vi "Test_Resize_Greyscale.vi"(8 "error in (no error)":errorcluster, 11 "Test Case In":refnum<class "Image.lvclass">) -> (0 "error out":errorcluster, 3 "Test Case Out":refnum<class "Image.lvclass">)   [LabVIEW 2020, in "g_ar_toolkit.test.lvlib" / "Image.lvclass"]
uses:
  Image.lvclass
  Image.lvclass/Image.ctl
  g_ar_toolkit.image/g_ar_toolkit.image.lvlib
  g_ar_toolkit.image/Image Size (Fixed).ctl
  g_ar_toolkit.image/CreateEmptyImageGreyscale.vi
  g_ar_toolkit.image/Interpolation Mode.ctl
  g_ar_toolkit.image/ResizeGreyscale.vi
  4993e8ee-a06a-463a-9684-69129f64d5ce.vi
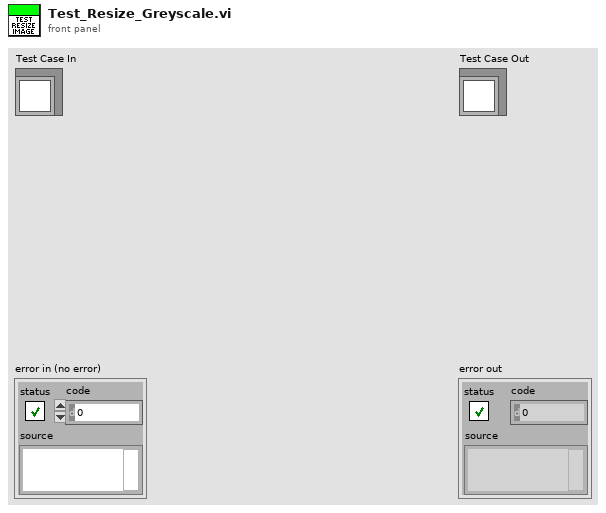
[diagram p1: front panel]
types:
  T1 = typedef "g_ar_toolkit.image.lvlib/Interpolation Mode.ctl" = enum8{"NEAREST", "LINEAR", "CUBIC", "AREA", "LANCZOS", "LINEAR_EXACT", "NEAREST_EXACT", "MAX"}
  T2 = typedef "g_ar_toolkit.image.lvlib/Image Size (Fixed).ctl" = cluster{"Width":u16, "Height":u16}
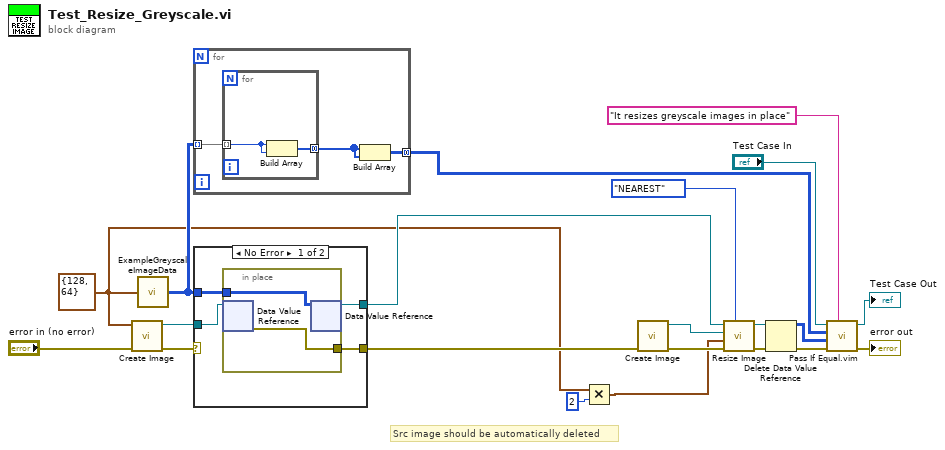
[diagram p0: block diagram]
diagram:
  w2 = T2 {"Width"=128, "Height"=64} ("Preallocated Image Size (Default - 0,0)")
  # "Src image should be automatically deleted"
  n1 = call-poly "Create Image.vi"("error in (no error)"="error in (no error)", "Preallocated Image Size (Default 0,0)"=w2) -> ("error out"=w15:errorcluster, "New Greyscale Image"=w14:refnum<data-value>)  [unwired: 8 in]
  n2 = call "ExampleGreyscaleImageData.vi"("Image Size"=w2) -> ("GreyscaleImage"=w8:u8[][])
  n3 = for {
    tunnel: w8 -> [w24] mode=indexing
    tunnel: [w22] -> w7 mode=concatenating
    n4 = for {
      tunnel: w24 -> [w26] mode=indexing
      tunnel: [w25] -> w23 mode=concatenating
      n5 = Build Array(w26, w26) -> (w25:u8[])
    }
    n6 = Build Array(w23, w23) -> (w22:u8[][])
  }
  n7 = case shown="No Error" w15 {
    selector: w15 -> [_ w33]
    tunnel: w14 -> [w30 w34]
    tunnel: w8 -> [w29 _]
    tunnel: [w28 w34] -> w12
    tunnel: [w27 w33] -> w5
    frame No Error {
      n8 = in-place {
        in-place-border: w29 -> [w32]
        in-place-border: [w31] -> w27
        n9 = in-place-dvr #1(w30) -> (w31:errorcluster)  [unwired: 1 out]
        n10 = in-place-dvr #1(w32) -> (w28:refnum<data-value>)  [unwired: 1 out]
      }
    }
    frame Error {
    }
  }
  n11 = Multiply(x=w2, y=u16 2) -> (x*y=w1:T2)
  n12 = call-poly "Create Image.vi"("error in (no error)"=w5) -> ("error out"=w4:errorcluster, "New Greyscale Image"=w3:refnum<data-value>)  [unwired: 9 in]
  n13 = call-poly "Resize Image.vi"("OpenCV Interpolation Flag"=Interpolation_Mode."NEAREST", "error in (no error)"=w4, "New Image Size"=w1, "Greyscale Destination Image"=w3, "Greyscale Source Image"=w12) -> ("error out"=w10:errorcluster, "Greyscale Destination Image (duplicate)"=w11:refnum<data-value>)  [unwired: 5 in]
  n14 = Delete Data Value Reference(data value reference=w11, error in=w10) -> (data value=w13:u8[][], error out=w17:errorcluster)
  n15 = call "Pass If Equal.vim"("Description"="It resizes greyscale images in place", "error in (no error)"=w17, "Actual"=w13, "Expected"=w7, "LUnit Test Case In"="Test Case In") -> ("error out"=→"error out":errorcluster, "LUnit Test Case Out"=→"Test Case Out":refnum<class "Image.lvclass">)  [unwired: 5 in]
